vi "U01_TCP_P2PREAD.vi"() -> ()   [LabVIEW 2015]
panel:
  in  "mode (standard)":T1(ring)
  in  "bytes to read":i32=4
  out "error out":errorcluster
  out "data out":string
  in  "service name IP":string
  in  "port":u16
  in  "timeout ms (wait forever: -1)":i32=-1
  in  "error in (no error)":errorcluster
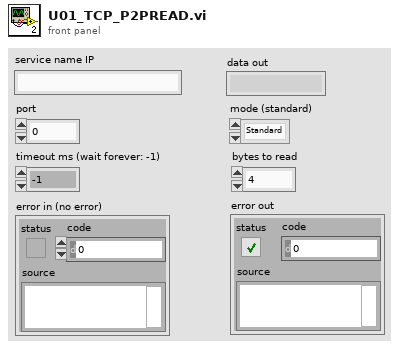
[diagram p1: front panel]
types:
  T1 = enum16{"Standard", "Buffered", "CRLF", "Immediate"}
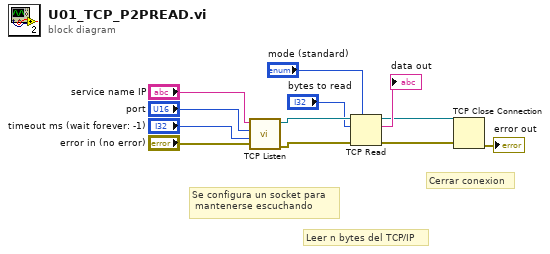
[diagram p0: block diagram]
diagram:
  # "Cerrar conexion"
  # "Leer n bytes del TCP/IP"
  # "Se configura un socket para\n mantenerse escuchando"
  n1 = call <vilib>:"TCP Listen.vi"("error in (no error)"="error in (no error)", "timeout ms (wait forever: -1)"="timeout ms (wait forever: -1)", "port"="port", "service name"="service name IP") -> ("error out"=w8:errorcluster, "connection ID"=w7:refnum<k5>)  [unwired: 3 in, 3 out]
  n2 = TCP Read(connection ID=w7, bytes to read="bytes to read", error in (no error)=w8, 7:"mode (standard)") -> (connection ID out=w3:refnum<k5>, data out=→"data out":string, error out=w4:errorcluster)  [unwired: 1 in]
  n3 = TCP Close Connection(connection ID=w3, error in (no error)=w4) -> (error out=→"error out":errorcluster)  [unwired: 1 in, 1 out]
